vi "EditParam2.vi"(11 "DevType":u32(ring)=4 items=["USB_CAN"=3, "USB_CAN2"=4]) -> (0 "InitConfig":T1, 1 "Chls":u32[](array[numeric]), 2 "DevIndex":u32, 3 "cancel":bool)   [LabVIEW 2011]
panel:
  in  "Cancel":bool
  in  "Ok":bool
  in  "mode":u16(ring) caption="工作模式：" items=["正常工作", "仅监帧听模式", "自测模试（环回模式）"]
  in  "Btr1":u8=20 caption="定时器1(BTR1)：0x" format="%02x"
  in  "Btr0":u8 caption="定时器0(BTR0)：0x" format="%02x"
  in  "BtrSelfdef":bool
  in  "br":u32(ring)=15 caption="波特率：" items=["10k bps"=2, "20k bps"=3, "40k bps"=4, "50k bps"=5, "80k bps"=6, "100k bps"=7, "125k bps"=8, "200k bps"=9, "250k bps"=10, "400k bps"=11, "500k bps"=12, "666k bps"=13, "800k bps"=14, "1000k bps"=15]
  in  "OpenAll":bool
  in  "Channel":u32(ring) caption="通道号：" items=["通道1", "通道2"]
  in  "DevInd":enum32{"0", "1", "2", "3", "4", "5", "6", "7"}(ring) caption="设备索引号："
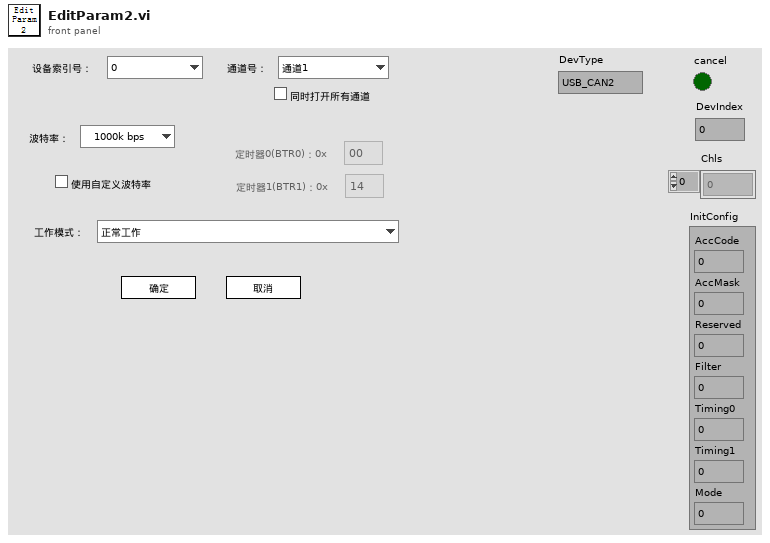
[diagram p1: front panel]
types:
  T1 = cluster{"AccCode":u32, "AccMask":u32, "Reserved":u32, "Filter":u8, "Timing0":u8, "Timing1":u8, "Mode":u8}
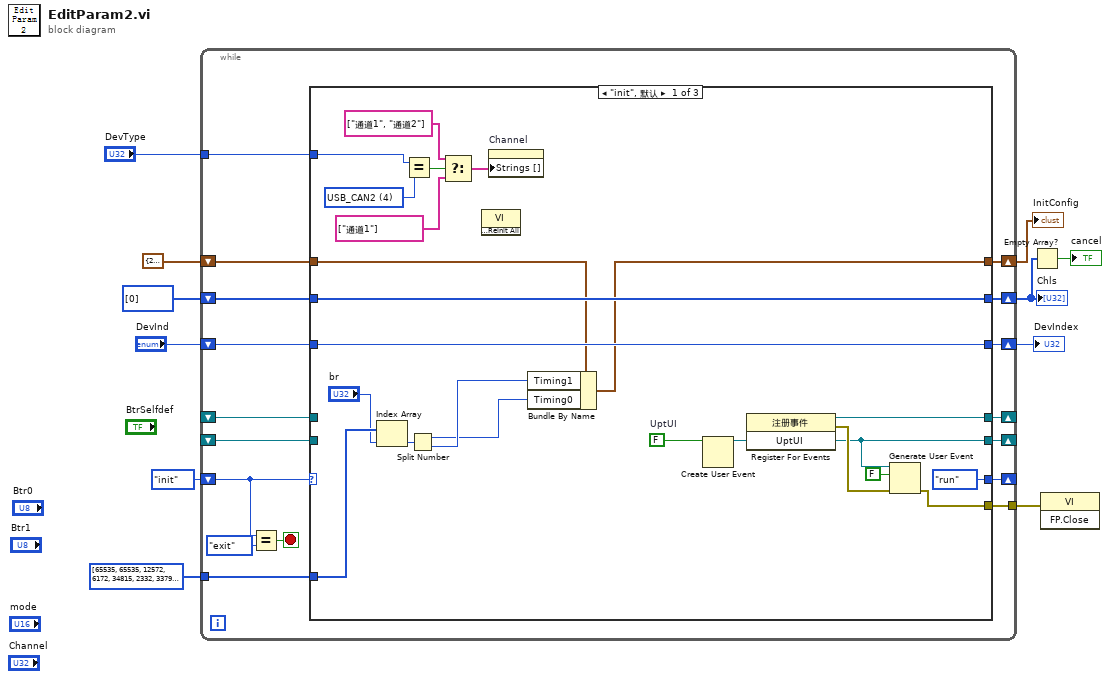
[diagram p0: block diagram]
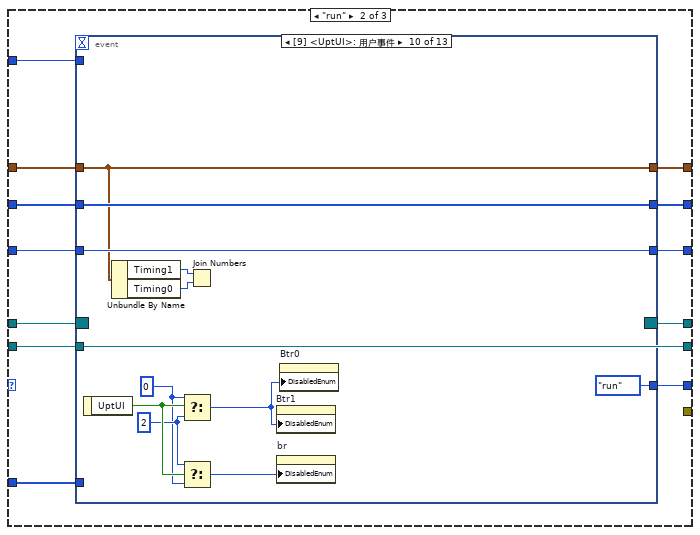
[diagram p2: hidden frame]
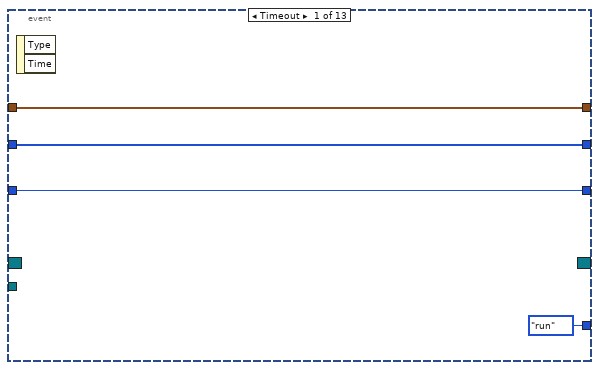
[diagram p3: hidden frame]
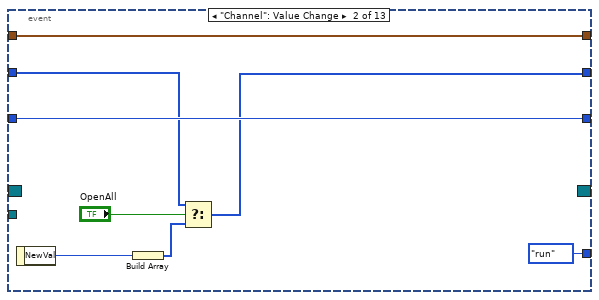
[diagram p4: hidden frame]
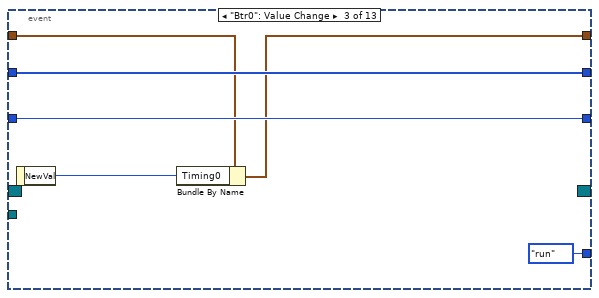
[diagram p5: hidden frame]
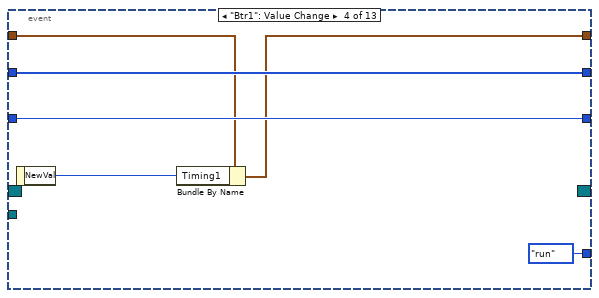
[diagram p6: hidden frame]
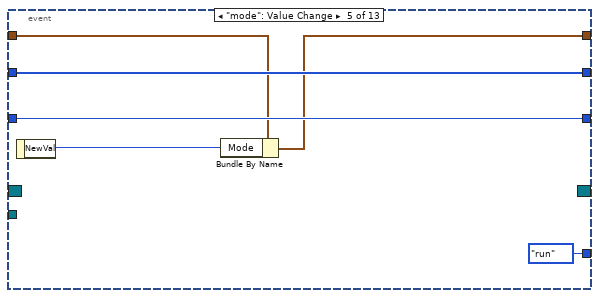
[diagram p7: hidden frame]
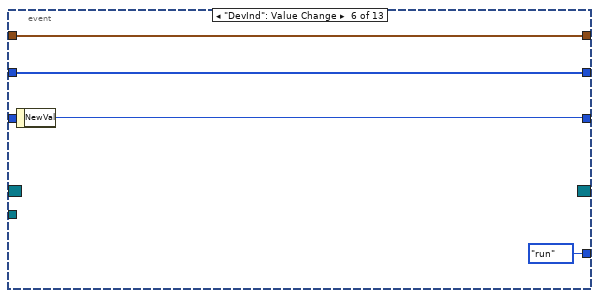
[diagram p8: hidden frame]
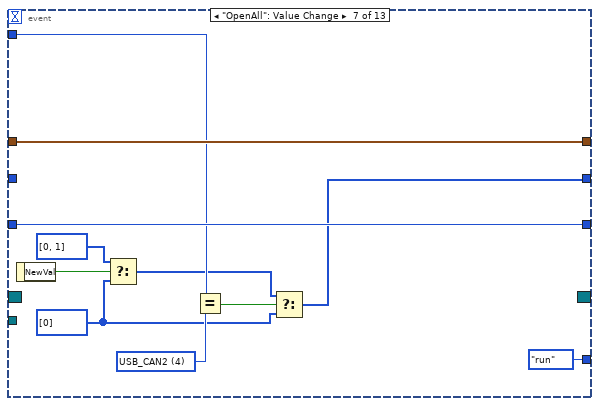
[diagram p9: hidden frame]
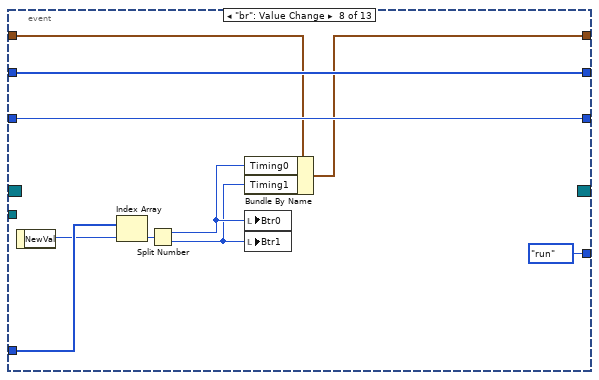
[diagram p10: hidden frame]
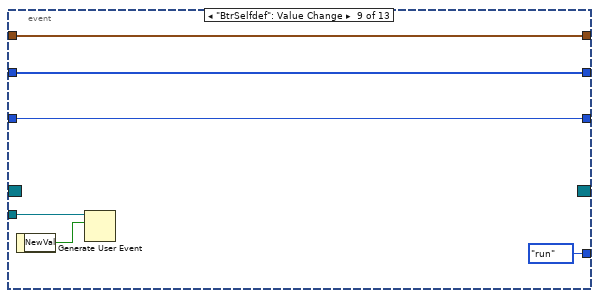
[diagram p11: hidden frame]
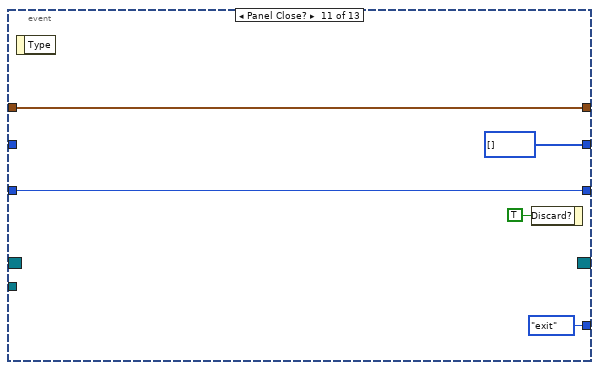
[diagram p12: hidden frame]
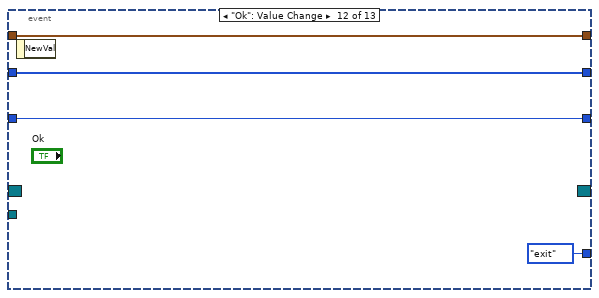
[diagram p13: hidden frame]
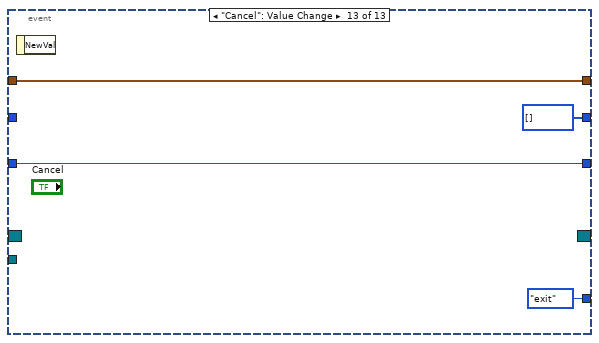
[diagram p14: hidden frame]
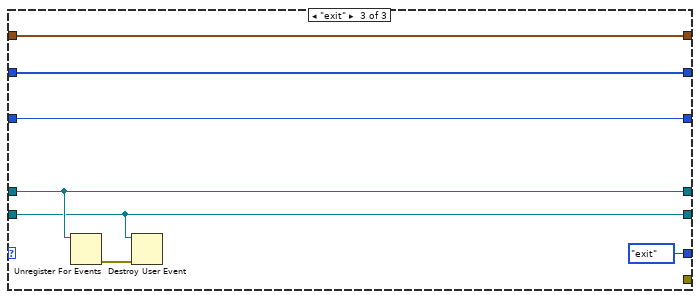
[diagram p15: hidden frame]
diagram:
  n1 = while {
    shift-right: [w25] -> _
    shift-left: enum16{"init", "run", "exit"}."init" -> [w26]
    tunnel: "DevType" -> [w24]
    shift-right: [w22] -> w5
    shift-left: T1 {"AccCode"=2147483656, "AccMask"=4294967295, "Reserved"=0, "Filter"=0, "Timing0"=0, "Timing1"=0, "Mode"=0} ("InitConfig") -> [w23]
    shift-right: [w20] -> w4
    shift-left: u32[] [0] ("Chls") -> [w21]
    shift-right: [w18] -> w6
    shift-left: "DevInd" -> [w19]
    shift-right: [w17] -> _
    shift-left: _ -> [w16]
    shift-right: [w15] -> _
    shift-left: _ -> [w14]
    tunnel: u16[] [65535, 65535, 12572, 6172, 34815, 2332, 33791, 1052, 796, 33274, 284, 33018, 28, 32950, 22, 20] ("Chls") -> [w13]
    tunnel: [w12] -> w1
    stop <- w27 stop-if-true
    n2 = Equal?(x=w26, y=enum16{"init", "run", "exit"}."exit") -> (x = y?=w27:bool)
    n3 = case shown="\"init\", 默认" w26 {
      tunnel: [enum16{"init", "run", "exit"}."run" w62 enum16{"init", "run", "exit"}."exit"] -> w25
      tunnel: w24 -> [w49 w51 _]
      tunnel: w23 -> [w33 w61 w154]
      tunnel: [w30 w60 w154] -> w22
      tunnel: w21 -> [w42 w59 w153]
      tunnel: [w42 w58 w153] -> w20
      tunnel: w19 -> [w41 w57 w152]
      tunnel: [w41 w56 w152] -> w18
      tunnel: [w40 w54 w150] -> w17
      tunnel: w16 -> [_ w55 w150]
      tunnel: [w38 w53 w148] -> w15
      tunnel: w14 -> [_ w53 w148]
      tunnel: w13 -> [w36 w52 _]
      tunnel: [w29 _ _] -> w12
      frame "init", Default {
        w43 = FALSE  # UptUI
        w48 = u32 4 items=["USB_CAN"=3, "USB_CAN2"=4] ("DevType")
        n4 = Index Array(array=w36, index="br") -> (element=w34:u16)
        n5 = Equal?(x=w49, y=w48) -> (x = y?=w47:bool)
        n6 = Split Number(x=w34) -> (hi(x)=w31:u8, lo(x)=w32:u8)
        n7 = Select(t=string[] ["通道1", "通道2"] ("字符串[]"), s=w47, f=string[] ["通道1"] ("字符串[]")) -> (s? t:f=w44:string[])
        n8 = invoke class="VI" method="Default Vals.Reinit All"() -> ()  [unwired: 3 in, 3 out]
        n9 = property on="Channel" class="Ring (严格)"("Strings []"=w44) -> ()  [unwired: 2 in, 2 out]
        n10 = Bundle By Name(cluster=w33, "Timing1"=w32, "Timing0"=w31) -> (w30:T1)
        n11 = Create User Event(user event datatype=w43) -> (user event=w38:refnum<user-event>)  [unwired: 1 in, 1 out]
        n12 = register-events(w38) -> (reference out=w40:refnum<event-registration>, error out=w39:errorcluster)  [unwired: 2 in]
        n13 = Generate User Event(user event=w38, event data cluster=FALSE ("事件数据"), error in=w39) -> (error out=w29:errorcluster)  [unwired: 1 out]
      }
      frame "run" {
        n14 = event shown="[9] <UptUI>: 用户事件" {
          selector: w55 -> [_ _ _ _ _ _ _ _ _ _ _ _ _]
          dyn-events: [_ _ _ _ _ _ _ _ _ _ _ _ _] -> w54
          timeout: _ -> [_ _ _ _ _ _ _ _ _ _ _ _ _]
          tunnel: [enum16{"init", "run", "exit"}."run" enum16{"init", "run", "exit"}."run" enum16{"init", "run", "exit"}."run" enum16{"init", "run", "exit"}."run" enum16{"init", "run", "exit"}."run" enum16{"init", "run", "exit"}."run" enum16{"init", "run", "exit"}."run" enum16{"init", "run", "exit"}."run" enum16{"init", "run", "exit"}."run" enum16{"init", "run", "exit"}."run" enum16{"init", "run", "exit"}."exit" enum16{"init", "run", "exit"}."exit" enum16{"init", "run", "exit"}."exit"] -> w62
          tunnel: w61 -> [w65 w73 w77 w83 w89 w95 w106 w111 w122 w131 w137 w142 w146]
          tunnel: [w65 w73 w75 w81 w87 w95 w106 w108 w122 w131 w137 w142 w146] -> w60
          tunnel: w59 -> [w64 w70 w79 w85 w91 w94 _ w116 w121 w133 _ w141 _]
          tunnel: [w64 w67 w79 w85 w91 w94 w97 w116 w121 w133 u32[] [] ("Chls") w141 u32[] [] ("Chls")] -> w58
          tunnel: w57 -> [w63 w72 w78 w84 w90 _ w105 w115 w120 w132 w136 w140 w145]
          tunnel: [w63 w72 w78 w84 w90 w93 w105 w115 w120 w132 w136 w140 w145] -> w56
          tunnel: w53 -> [_ _ _ _ _ _ _ _ w119 _ _ _ _]
          tunnel: w52 -> [_ _ _ _ _ _ _ w113 _ _ _ _ _]
          tunnel: w51 -> [_ _ _ _ _ _ w104 _ _ _ _ _ _]
          event Timeout {
            n15 = event-data() -> ()  [unwired: 1 in, 2 out]
          }
          event "Channel": Value Change {
            n16 = event-data() -> ("NewVal"=w69:u32)  [unwired: 1 in]
            n17 = Build Array(w69) -> (w68:u32[])
            n18 = Select(t=w70, s="OpenAll", f=w68) -> (s? t:f=w67:u32[])
          }
          event "Btr0": Value Change {
            n19 = event-data() -> ("NewVal"=w76:u8)  [unwired: 1 in]
            n20 = Bundle By Name(cluster=w77, "Timing0"=w76) -> (w75:T1)
          }
          event "Btr1": Value Change {
            n21 = event-data() -> ("NewVal"=w82:u8)  [unwired: 1 in]
            n22 = Bundle By Name(cluster=w83, "Timing1"=w82) -> (w81:T1)
          }
          event "mode": Value Change {
            n23 = event-data() -> ("NewVal"=w88:u16)  [unwired: 1 in]
            n24 = Bundle By Name(cluster=w89, "Mode"=w88) -> (w87:T1)
          }
          event "DevInd": Value Change {
            n25 = event-data() -> ("NewVal"=w93:enum32{"0", "1", "2", "3", "4", "5", "6", "7"})  [unwired: 1 in]
          }
          event "OpenAll": Value Change {
            w98 = u32[] [0] ("Chls")
            w103 = u32 4 items=["USB_CAN"=3, "USB_CAN2"=4] ("DevType")
            n26 = event-data() -> ("NewVal"=w101:bool)  [unwired: 1 in]
            n27 = Select(t=u32[] [0, 1] ("Chls"), s=w101, f=w98) -> (s? t:f=w99:u32[])
            n28 = Equal?(x=w104, y=w103) -> (x = y?=w102:bool)
            n29 = Select(t=w99, s=w102, f=w98) -> (s? t:f=w97:u32[])
          }
          event "br": Value Change {
            n30 = event-data() -> ("NewVal"=w112:u32)  [unwired: 1 in]
            n31 = Index Array(array=w113, index=w112) -> (element=w114:u16)
            n32 = Split Number(x=w114) -> (hi(x)=w110:u8, lo(x)=w109:u8)
            n33 = Bundle By Name(cluster=w111, "Timing0"=w110, "Timing1"=w109) -> (w108:T1)
            n34 = local write "Btr0"(w110) -> ()
            n35 = local write "Btr1"(w109) -> ()
          }
          event "BtrSelfdef": Value Change {
            n36 = event-data() -> ("NewVal"=w118:bool)  [unwired: 1 in]
            n37 = Generate User Event(user event=w119, event data cluster=w118) -> ()  [unwired: 1 in, 2 out]
          }
          event User Event {
            w126 = 2
            w125 = 0
            n38 = event-data() -> ("UptUI"=w127:bool)  [unwired: 1 in]
            n39 = Unbundle By Name(w131) -> ("Timing1"=w129:u8, "Timing0"=w130:u8)
            n40 = Select(t=w125, s=w127, f=w126) -> (s? t:f=w128:i32)
            n41 = Select(t=w126, s=w127, f=w125) -> (s? t:f=w124:i32)
            n42 = Join Numbers(hi=w129, lo=w130) -> ()  [unwired: 1 out]
            n43 = property on="Btr1" class="DigNum (严格)"("DisabledEnum"=w128) -> ()  [unwired: 2 in, 2 out]
            n44 = property on="br" class="Ring (严格)"("DisabledEnum"=w124) -> ()  [unwired: 2 in, 2 out]
            n45 = property on="Btr0" class="DigNum (严格)"("DisabledEnum"=w128) -> ()  [unwired: 2 in, 2 out]
          }
          event Panel Close? {
            n46 = event-data() -> ()  [unwired: 1 in, 1 out]
            n47 = event-data("Discard?"=TRUE ("放弃？")) -> ()  [unwired: 1 in, 1 out]
          }
          event "Ok": Value Change {
            n48 = event-data() -> ()  [unwired: 1 in, 1 out]
          }
          event "Cancel": Value Change {
            n49 = event-data() -> ()  [unwired: 1 in, 1 out]
          }
        }
      }
      frame "exit" {
        n50 = Unregister For Events(event registration refnum=w150) -> (error out=w149:errorcluster)  [unwired: 1 in]
        n51 = Destroy User Event(user event=w148, error in=w149) -> ()  [unwired: 1 out]
      }
    }
  }
  "DevIndex" <- w6
  "Chls" <- w4
  "InitConfig" <- w5
  n52 = Empty Array?(array=w4) -> (empty?=→"cancel":bool)
  n53 = invoke class="VI" method="FP.Close"(error in=w1) -> ()  [unwired: 2 in, 3 out]
